vi "Fetch Measurement (Multiple Points).vi"(8 "error in (no error)":errorcluster, 9 "Data Mode (5: Voltage)":i32(ring)=5 items=["Current", "Resistance", "Source Output Setting", "Status", "Time", "Voltage"], 10 "Channel (0: Channel 1)":i32(ring) items=["Channel 1", "Channel 2"], 11 "VISA resource name":refnum<visa-resource-name>) -> (0 "error out":errorcluster, 2 "Measurements":dbl[](array[numeric]), 3 "VISA resource name out":refnum<visa-resource-name>)   [LabVIEW 2023, in "Agilent B2900 Series.lvlib"]
doc: "Returns the array data which contains all data of the voltage measurement, current measurement, resistance measurement data, time, status, or source output setting.\n\n<B>Note:</B> Use this VI only with other low-level VIs. The high-level VIs automatically incorporate this functionality. This VI does not check the instrument status."
uses:
  Agilent B2900 Series.lvlib
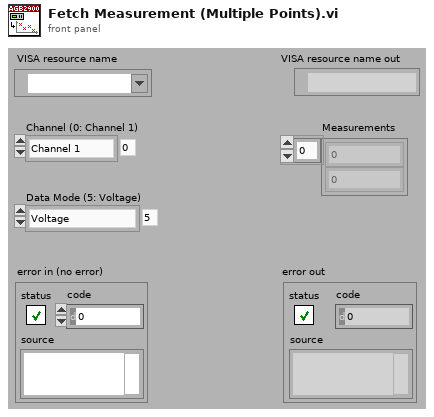
[diagram p1: front panel]
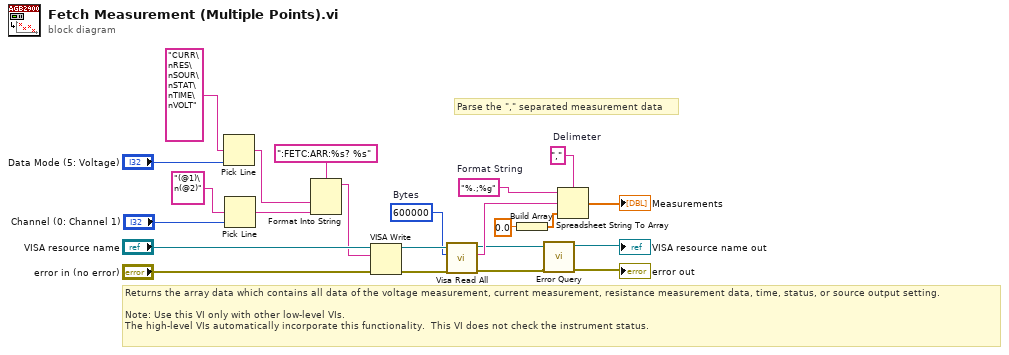
[diagram p0: block diagram]
diagram:
  w9 = u32 600000  # Bytes
  w11 = ","  # Delimeter
  w16 = "%.;%g"  # Format String
  # "Returns the array data which contains all data of the voltage measurement, current measurement, resistance measurement data, time, status, or source output setting.\n\nNote: Use this VI only with other low-level VIs.  \nThe high-level VIs automatically incorporate this functionality.  This VI does not check the instrument status."
  # "Parse the \",\" separated measurement data"
  n1 = Pick Line(multi-line string="CURR\nRES\nSOUR\nSTAT\nTIME\nVOLT", line index="Data Mode (5: Voltage)") -> (output string=w8:string)  [unwired: 1 in]
  n2 = Pick Line(multi-line string="(@1)\n(@2)", line index="Channel (0: Channel 1)") -> (output string=w5:string)  [unwired: 1 in]
  n3 = Format Into String(format string=":FETC:ARR:%s? %s", w8, w5) -> (resulting string=w10:string)  [unwired: 2 in, 1 out]
  n4 = VISA Write(VISA resource name="VISA resource name", write buffer=w10, error in (no error)="error in (no error)") -> (VISA resource name out=w18:refnum<visa-resource-name>, error out=w17:errorcluster)  [unwired: 1 out]
  n5 = call "Visa Read All.vi"("error in (no error)"=w17, "Byte Count Each Loop (6000)"=w9, "VISA resource name"=w18) -> ("error out"=w3:errorcluster, "Read Buffer"=w15:string, "VISA resource name out"=w4:refnum<visa-resource-name>)  [unwired: 6 in]
  n6 = Build Array(0.0) -> (w14:dbl[])
  n7 = call "Error Query.vi"("error in (no error)"=w3, "VISA resource name"=w4) -> ("error out"=→"error out":errorcluster, "VISA resource name out"=→"VISA resource name out":refnum<visa-resource-name>)  [unwired: 6 in, 2 out]
  n8 = Spreadsheet String To Array(delimiter (Tab)=w11, format string=w16, spreadsheet string=w15, array type (2D Dbl)=w14) -> (array=→"Measurements":dbl[])
